vi "cast_to_Interface.vi"(1 "Object":refnum<class>, 3 "method refs":T1, 5 "error in (no error)":errorcluster) -> (14 "Interface_object out":refnum<class "DoorInterface.lvclass">, 19 "error out":errorcluster)   [LabVIEW 2018, in "DoorInterface.lvclass"]
doc: "Casts object to type of the interface and assign static method references. This method must be called only from corresponding methods belonging to the interface-applying classes."
uses:
  DoorInterface.lvclass
  method_refs.ctl
  DoorInterface.lvclass/DoorInterface.ctl
panel:
  # "Do not edit this method"
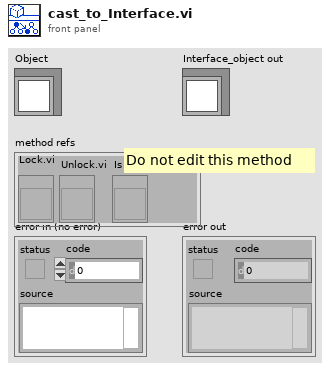
[diagram p1: front panel]
types:
  T1 = typedef "DoorInterface.lvclass/method_refs.ctl" = cluster{"Lock.vi":refnum<vi>, "Unlock.vi":refnum<vi>, "Is Door Open.vi":refnum<vi>}
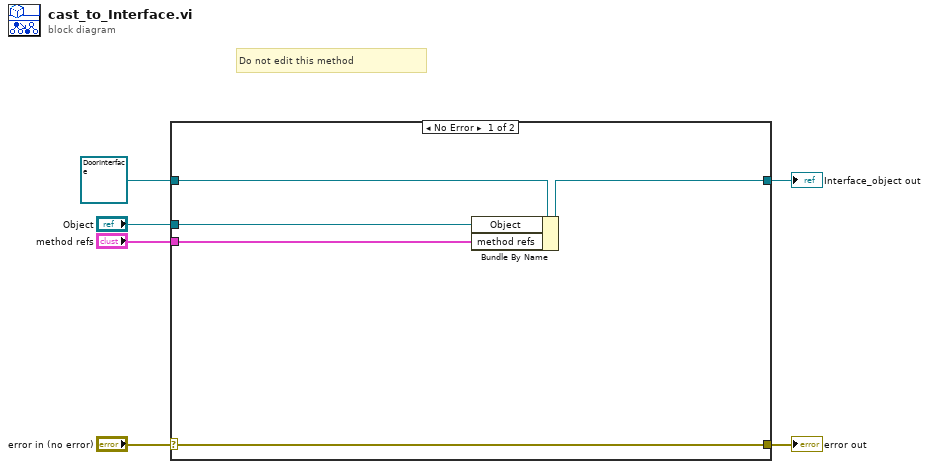
[diagram p0: block diagram]
diagram:
  # "Do not edit this method"
  n1 = case shown="No Error" "error in (no error)" {
    selector: "error in (no error)" -> [w10 w13]
    tunnel: [w10 w13] -> w5
    tunnel: [w9 w12] -> w3
    tunnel: refnum<class "DoorInterface.lvclass"> refnum ("AZ_Interface_Template in") -> [w11 w12]
    tunnel: "Object" -> [w8 _]
    tunnel: "method refs" -> [w7 _]
    frame No Error {
      n2 = Bundle By Name(cluster=w11, "Object"=w8, "method refs"=w7) -> (w9:refnum<class "DoorInterface.lvclass">)
    }
    frame Error {
    }
  }
  "error out" <- w5
  "Interface_object out" <- w3
